vi "toString.vi"(11 "Telemetry":T1) -> (3 "String":string)   [LabVIEW 2012]
uses:
  Formula Hybrid 2012 r1/Telemetry.ctl
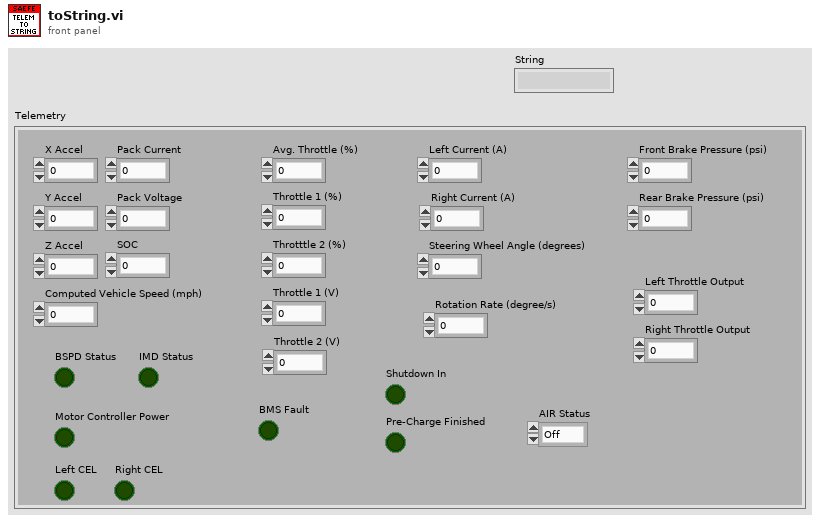
[diagram p1: front panel]
types:
  T1 = typedef "Telemetry.ctl" = cluster{"X Accel":dbl, "Y Accel":dbl, "Pack Current":dbl, "Pack Voltage":dbl, "SOC":dbl, "Avg. Throttle (%)":dbl, "Z Accel":dbl, "Throttle 1 (%)":dbl, "Throtttle 2 (%)":dbl, "Throttle 1 (V)":dbl, "Throttle 2 (V)":dbl, "Left Current (A)":dbl, "Right Current (A)":dbl, "Steering Wheel Angle (degrees)":dbl, "Rotation Rate (degree/s)":dbl, "Front Brake Pressure (psi)":dbl, "Rear Brake Pressure (psi)":dbl, "Computed Vehicle Speed (mph)":dbl, "BSPD Status":bool, "IMD Status":bool, "Motor Controller Power":bool, "Left CEL":bool, "Right CEL":bool, "BMS Fault":bool, "Shutdown In":bool, "Pre-Charge Finished":bool, "AIR Status":enum16{"Off", "Precharge", "On"}, "Left Throttle Output":fxp<+/-,20,7>, "Right Throttle Output":fxp<+/-,20,7>}
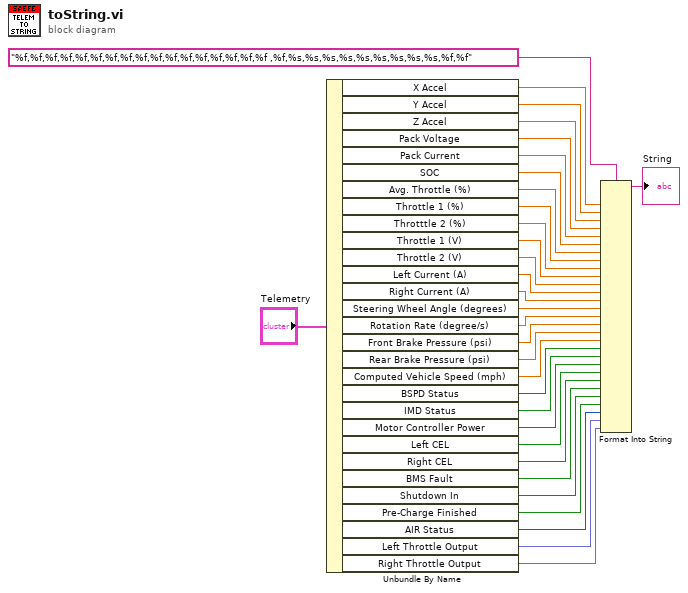
[diagram p0: block diagram]
diagram:
  n1 = Unbundle By Name("Telemetry") -> ("X Accel"=w31:dbl, "Y Accel"=w30:dbl, "Z Accel"=w29:dbl, "Pack Voltage"=w28:dbl, "Pack Current"=w27:dbl, "SOC"=w26:dbl, "Avg. Throttle (%)"=w25:dbl, "Throttle 1 (%)"=w24:dbl, "Throtttle 2 (%)"=w23:dbl, "Throttle 1 (V)"=w22:dbl, "Throttle 2 (V)"=w21:dbl, "Left Current (A)"=w20:dbl, "Right Current (A)"=w19:dbl, "Steering Wheel Angle (degrees)"=w18:dbl, "Rotation Rate (degree/s)"=w17:dbl, "Front Brake Pressure (psi)"=w16:dbl, "Rear Brake Pressure (psi)"=w15:dbl, "Computed Vehicle Speed (mph)"=w14:dbl, "BSPD Status"=w13:bool, "IMD Status"=w12:bool, "Motor Controller Power"=w11:bool, "Left CEL"=w10:bool, "Right CEL"=w9:bool, "BMS Fault"=w8:bool, "Shutdown In"=w7:bool, "Pre-Charge Finished"=w6:bool, "AIR Status"=w5:enum16{"Off", "Precharge", "On"}, "Left Throttle Output"=w1:fxp<+/-,20,7>, "Right Throttle Output"=w2:fxp<+/-,20,7>)
  n2 = Format Into String(format string="%f,%f,%f,%f,%f,%f,%f,%f,%f,%f,%f,%f,%f,%f,%f,%f,%f ,%f,%s,%s,%s,%s,%s,%s,%s,%s,%s,%f,%f", w31, w30, w29, w28, w27, w26, w25, w24, w23, w22, w21, w20, w19, w18, w17, w16, w15, w14, w13, w12, w11, w10, w9, w8, w7, w6, w5, w1, w2) -> (resulting string=→"String":string)  [unwired: 2 in, 1 out]
